vi "Change Decoration Color.vi"(8 "error in (no error)":errorcluster, 11 "Decoration Color":u32(colorbox)) -> (0 "error out":errorcluster)   [LabVIEW 2017]
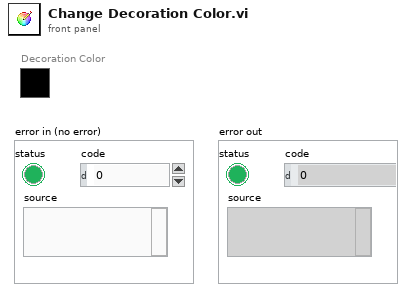
[diagram p1: front panel]
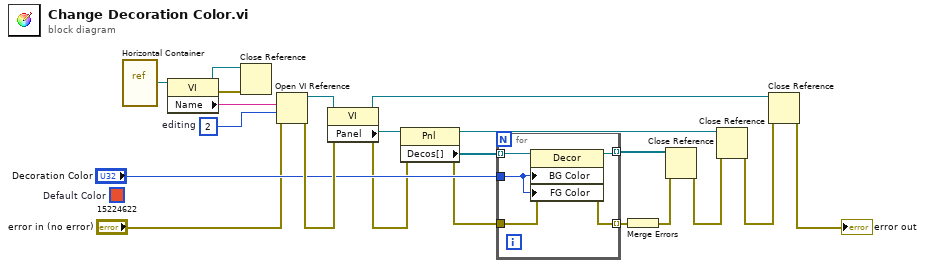
[diagram p0: block diagram]
diagram:
  (unwired) u32 15224622  # Default Color
  w19 = 2  # editing
  n1 = vi-ref "Horizontal Container.vi"() -> (w21:refnum<vi>)
  n2 = property class="VI"(reference=w21) -> (reference out=w7:refnum<vi>, error out=w8:errorcluster, "Name"=w20:string)  [unwired: 1 in]
  n3 = Close Reference(reference=w7, error in (no error)=w8) -> ()  [unwired: 1 out]
  n4 = Open VI Reference(vi path=w20, options=w19, error in (no error)="error in (no error)") -> (vi reference=w18:refnum<vi>, error out=w17:errorcluster)  [unwired: 3 in]
  n5 = property class="VI"(reference=w18, error in=w17) -> (reference out=w9:refnum<vi>, error out=w3:errorcluster, "Panel"=w16:refnum<vi>)
  n6 = property class="Pnl"(reference=w16, error in=w3) -> (reference out=w12:refnum<vi>, error out=w2:errorcluster, "Decos[]"=w15:refnum<vi>[])
  n7 = for {
    tunnel: w15 -> [w26] mode=indexing
    tunnel: "Decoration Color" -> [w24]
    tunnel: [w25] -> w13 mode=indexing
    tunnel: [w23] -> w5 mode=indexing
    tunnel: w2 -> [w22]
    n8 = property class="Decor"(reference=w26, error in=w22, "BG Color"=w24, "FG Color"=w24) -> (reference out=w25:refnum<vi>, error out=w23:errorcluster)
  }
  n9 = Merge Errors(w5) -> (w4:errorcluster)
  n10 = Close Reference(reference=w13, error in (no error)=w4) -> (error out=w11:errorcluster)
  n11 = Close Reference(reference=w12, error in (no error)=w11) -> (error out=w10:errorcluster)
  n12 = Close Reference(reference=w9, error in (no error)=w10) -> (error out=→"error out":errorcluster)
